vi "GEA2 Board ID to Board Index.vi"(0 "Board ID":string, 11 "Error In":errorcluster) -> (4 "Board Found?":bool, 6 "Report Text":string="Board not found.", 8 "Board Index":i32=-1, 10 "Boards Found":string[](array[string]), 15 "Error Out":errorcluster)   [LabVIEW 2016, in "GEA2_Toolkit.lvlib"]
doc: "This VI should be placed before the GEA2 Initialize VI. This VI will output the corresponding GEA2 bus index for a given NewFI board ID input."
uses:
  library/GEA2_Toolkit.lvlib
  C:/Technology Lab/NI-2010/Trunk/Utility/LabVIEW GEA2 Toolkit v1.0.0.0/Appliance.NET/GeaCommunication.Usb.dll
  Appliance.NET/GeaCommunication.Usb.dll
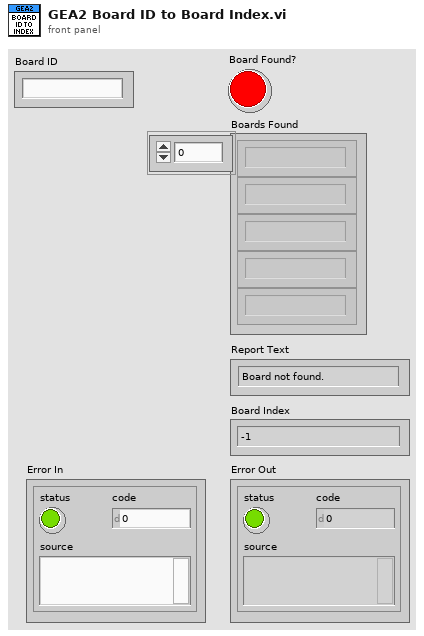
[diagram p1: front panel]
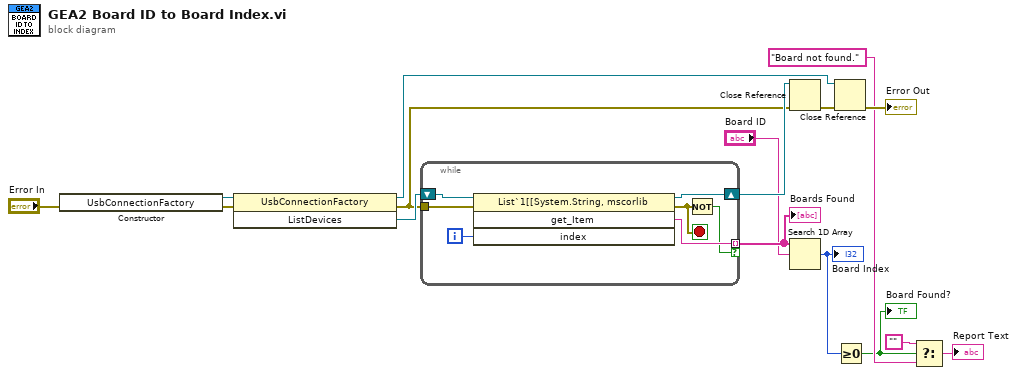
[diagram p0: block diagram]
diagram:
  n1 = constructor class="UsbConnectionFactory"(error in="Error In") -> (reference out=w16:refnum<k24>, error out=w15:errorcluster)  [unwired: 2 in, 1 out]
  n2 = invoke class="UsbConnectionFactory" method="ListDevices"(reference=w16, error in=w15) -> (reference out=w10:refnum<k24>, error out=w9:errorcluster, "ListDevices"=w14:refnum<k24>)  [unwired: 1 in]
  n3 = while {
    shift-right: [w22] -> w11
    shift-left: w14 -> [w23]
    tunnel: w9 -> [w20]
    tunnel: [w19] -> w4 mode=indexing if=w17
    i -> [w21]
    stop <- w18 stop-if-true
    n4 = invoke class="List`1[[System.String, mscorlib" method="get_Item"(reference=w23, error in=w20, "index"=w21) -> (reference out=w22:refnum<k24>, error out=w18:errorcluster, "get_Item"=w19:string)  [unwired: 1 in, 1 out]
    n5 = Not(x=w18) -> (.not. x?=w17:bool)
  }
  "Boards Found" <- w4
  n6 = Close Reference(reference=w11, error in (no error)=w9) -> (error out=w12:errorcluster)
  n7 = Search 1D Array(1D array=w4, element="Board ID") -> (index of element=w2:i32)  [unwired: 1 in]
  "Board Index" <- w2
  n8 = Close Reference(reference=w10, error in (no error)=w12) -> (error out=→"Error Out":errorcluster)
  n9 = Greater Or Equal To 0?(x=w2) -> (x >= 0?=w1:bool)
  "Board Found?" <- w1
  n10 = Select(t="", s=w1, f="Board not found.") -> (s? t:f=→"Report Text":string)
